vi "GetOptimalDFTSize.vi"(8 "error in":errorcluster, 11 "vecsize":i32) -> (0 "error out":errorcluster, 3 "OptimalSize":i32)   [LabVIEW 2020, in "OpenLvVision_OpenCv.lvlib"]
doc: "Returns the optimal DFT size for a given vector size. \n\nDFT performance is not a monotonic function of a vector size. Therefore, when you calculate convolution of two arrays or perform the spectral analysis of an array, it usually makes sense to pad the input data with zeros to get a bit larger array that can be transformed much faster than the original one. Arrays whose size is a power-of-two (2, 4, 8, 16, 32, ...) are the fastest to process. Though, the arrays whose size is a product of 2's, 3's, and 5's (for example, 300 = 5*5*3*2*2) are also processed quite efficiently."
uses:
  OpenLvVision_OpenCv.lvlib
  Dlls/OlvOpenCvWrapper.dll
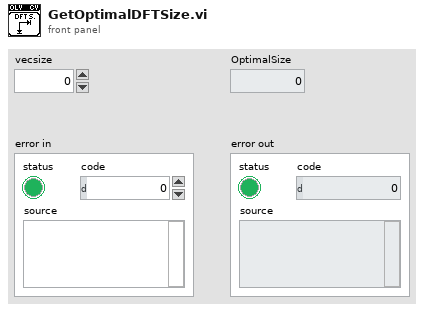
[diagram p1: front panel]
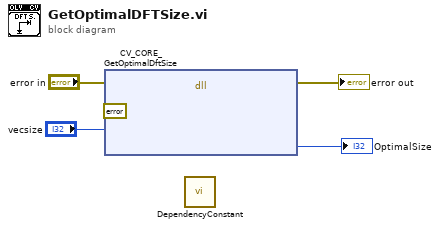
[diagram p0: block diagram]
diagram:
  n1 = dll-call lib="C:/Users/lukas/Downloads/OpenLvVision_OpenCv/SourceCode/LabView/OpenLvVision_OpenCv/Dlls/OlvOpenCvWrapper.dll" fn="CV_CORE_GetOptimalDftSize"(error in="error in", "Error"=errorcluster {"status"=FALSE, "code"=0, "source"=""} ("error constant"), "vecsize"="vecsize") -> (error out=→"error out":errorcluster, "optimalSizeOut"=→"OptimalSize":i32)  [unwired: 6 in, 1 out]
  n2 = call "DependencyConstant.vi"() -> ()  [unwired: 12 in]
